vi "Continuous Buffered Acquisition with Logging.vi"() -> ()   [LabVIEW 2009]
uses:
  <vilib>/DAQmx/configure/timing.llb/DAQmx Timing (Sample Clock).vi
  <vilib>/DAQmx/create/channels.llb/DAQmx Create Channel (AI-Voltage-Basic).vi
  <vilib>/DAQmx/read.llb/DAQmx Read (Analog Wfm 1Chan NSamp).vi
panel:
  out "data":waveform(dbl)(graph)
  in  "stop":bool
  in  "rate":dbl=1000.0 format="%0.2f"
  in  "physical channels":tag
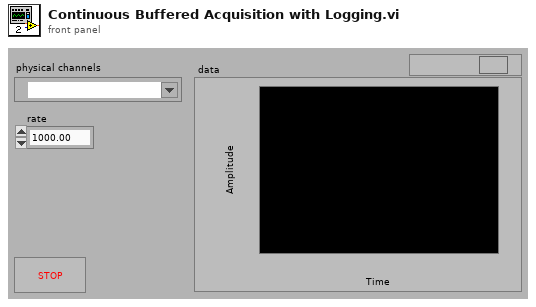
[diagram p1: front panel]
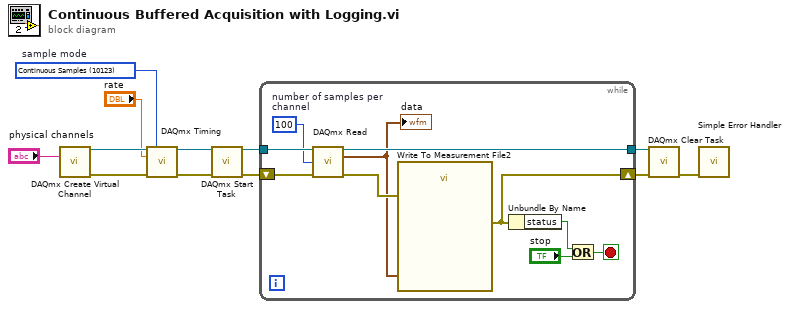
[diagram p0: block diagram]
diagram:
  w4 = 10123 items=["Finite Samples"=10178, "Continuous Samples"=10123, "Hardware Timed Single Point"=12522]  # sample mode
  n1 = call-poly <vilib>:"DAQmx Create Virtual Channel.vi"("physical channels"="physical channels") -> ("task out"=w9:refnum<k21>, "error out"=w6:errorcluster)  [unwired: 13 in]
  n2 = call-poly <vilib>:"DAQmx Timing.vi"("task/channels in"=w9, "sample mode"=w4, "rate"="rate", "error in"=w6) -> ("task out"=w8:refnum<k21>, "error out"=w7:errorcluster)  [unwired: 10 in]
  n3 = call <vilib>:"DAQmx Start Task.vi"("task/channels in"=w8, "error in"=w7) -> ("task out"=w3:refnum<k21>, "error out"=w2:errorcluster)  [unwired: 12 in]
  n4 = while {
    tunnel: [w17] -> w10
    tunnel: w3 -> [w21]
    shift-right: [w15] -> w12
    shift-left: w2 -> [w22]
    stop <- w20 stop-if-true
    w14 = 100  # number of samples per channel
    n5 = call-poly <vilib>:"DAQmx Read.vi"("task/channels in"=w21, "number of samples per channel"=w14, "error in"=w22) -> ("task out"=w17:refnum<k21>, "data"=w13:waveform(dbl), "error out"=w16:errorcluster)  [unwired: 10 in]
    "data" <- w13
    n6 = call "Write To Measurement File2"("Signals"=w13, "error in (no error)"=w16) -> ("error out"=w15:errorcluster)  [unwired: 15 in, 2 out]
    n7 = Unbundle By Name "Unbundle By Name"(w15) -> ("status"=w19:bool)
    n8 = Or(x=w19, y="stop") -> (x .or. y?=w20:bool)
  }
  n9 = call <vilib>:"DAQmx Clear Task.vi"("task in"=w10, "error in"=w12) -> ("error out"=w11:errorcluster)  [unwired: 13 in]
  n10 = call <vilib>:"Simple Error Handler.vi"("error in (no error)"=w11) -> ()  [unwired: 4 in, 5 out]
